vi "Meas Proc QWTB Fix Result Table Selection.vi"(7 "param table ref":refnum<vi>, 8 "error in":errorcluster) -> (0 "error out":errorcluster)   [LabVIEW 2013]
doc: "Detects position of the curcor in the table and sets selection to whole row accordingly."
uses:
  <vilib>/Utility/miscctls.llb/LVRowAndColumnTypeDef.ctl
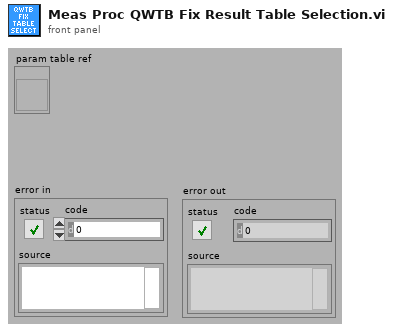
[diagram p1: front panel]
types:
  T1 = typedef "LVRowAndColumnTypeDef.ctl" = cluster{"Row":i32, "Column":i32}
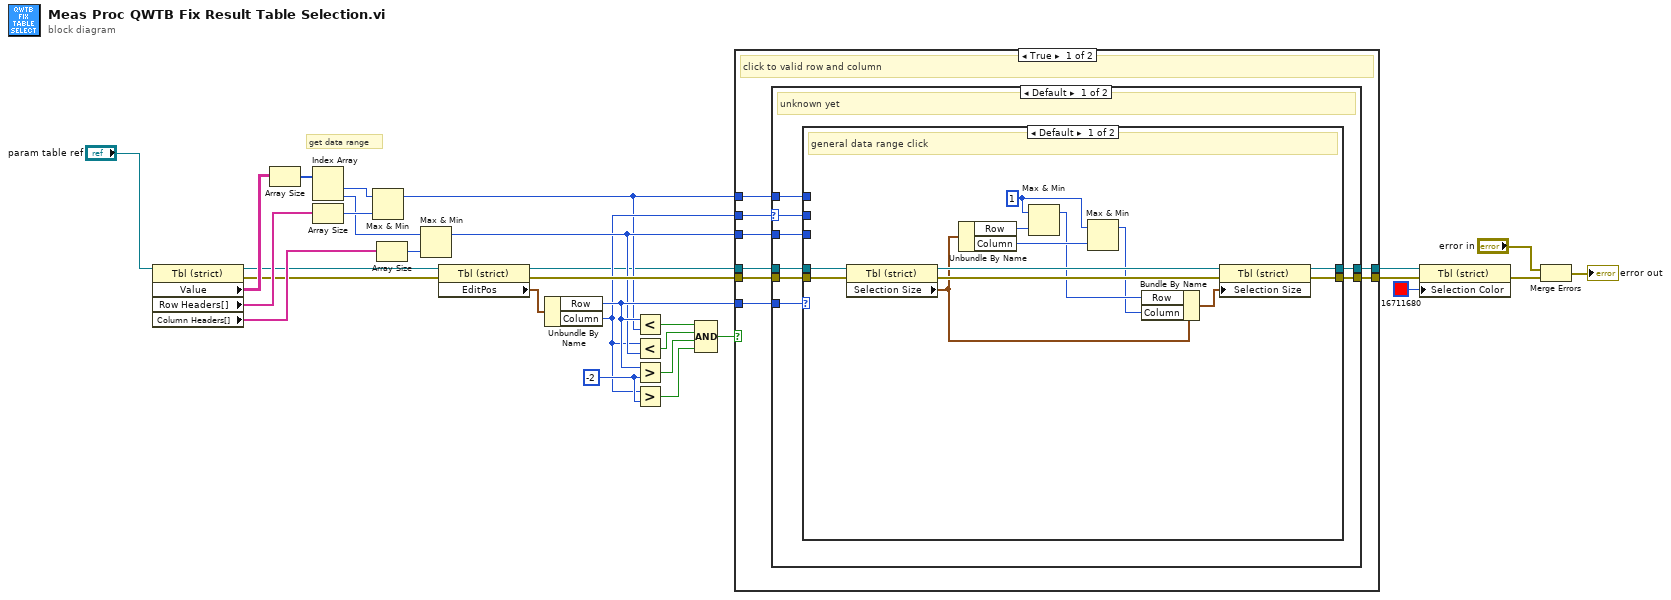
[diagram p0: block diagram]
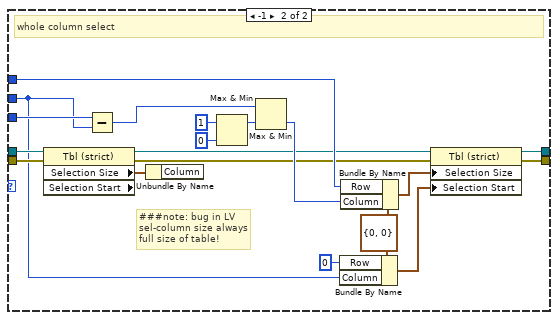
[diagram p2: hidden frame]
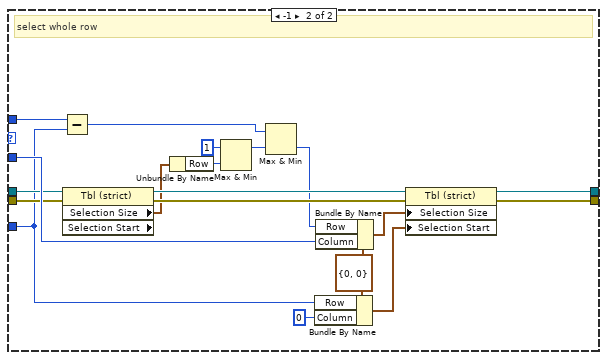
[diagram p3: hidden frame]
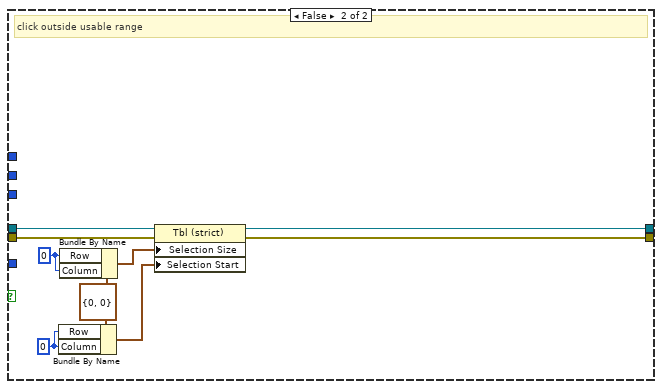
[diagram p4: hidden frame]
diagram:
  w10 = -2 ("y")
  # "get data range"
  n1 = property class="Tbl (strict)"(reference="param table ref") -> (reference out=w21:refnum<vi>, error out=w19:errorcluster, "Value"=w28:string[][], "Row Headers[]"=w26:string[], "Column Headers[]"=w22:string[])  [unwired: 1 in]
  n2 = Array Size(array=w28) -> (size(s)=w27:i32[])
  n3 = Index Array(array=w27) -> (element #1=w3:i32, element #2=w2:i32)  [unwired: 2 in]
  n4 = Array Size(array=w26) -> (size(s)=w25:i32)
  n5 = Max & Min(x=w3, y=w25) -> (max(x,y)=w4:i32)  [unwired: 1 out]
  n6 = Array Size(array=w22) -> (size(s)=w23:i32)
  n7 = Max & Min(x=w2, y=w23) -> (max(x,y)=w6:i32)  [unwired: 1 out]
  n8 = property class="Tbl (strict)"(reference=w21, error in=w19) -> (reference out=w1:refnum<vi>, error out=w18:errorcluster, "EditPos"=w20:T1)
  n9 = Unbundle By Name(w20) -> ("Row"=w11:i32, "Column"=w5:i32)
  n10 = Less?(x=w11, y=w4) -> (x < y?=w13:bool)
  n11 = Less?(x=w5, y=w6) -> (x < y?=w12:bool)
  n12 = Greater?(x=w11, y=w10) -> (0:w9:bool)
  n13 = Greater?(x=w5, y=w10) -> (0:w8:bool)
  n14 = Compound Arithmetic op=AND(w13, w12, w9, w8) -> (w7:bool)
  n15 = case shown="True" w7 {
    tunnel: w18 -> [w38 w106]
    tunnel: w1 -> [w37 w105]
    tunnel: w11 -> [w33 _]
    tunnel: w6 -> [w36 _]
    tunnel: [w35 w101] -> w17
    tunnel: [w34 w100] -> w16
    tunnel: w5 -> [w32 _]
    tunnel: w4 -> [w31 _]
    frame True {
      # "click to valid row and column"
      n16 = case shown="Default" w32 {
        selector: w32 -> [w40 _]
        tunnel: w38 -> [w46 w90]
        tunnel: w37 -> [w45 w89]
        tunnel: w36 -> [w44 w96]
        tunnel: [w43 w92] -> w35
        tunnel: [w42 w91] -> w34
        tunnel: w33 -> [w41 w82]
        tunnel: w31 -> [w39 w83]
        frame Default {
          # "unknown yet"
          n17 = case shown="Default" w41 {
            tunnel: w46 -> [w59 w72]
            tunnel: w45 -> [w58 w71]
            tunnel: w44 -> [_ w70]
            tunnel: [w55 w74] -> w43
            tunnel: [w54 w73] -> w42
            tunnel: w40 -> [_ w65]
            tunnel: w39 -> [_ w63]
            frame Default {
              w51 = 1 ("x")
              # "general data range click"
              n18 = property class="Tbl (strict)"(reference=w58, error in=w59) -> (reference out=w56:refnum<vi>, error out=w57:errorcluster, "Selection Size"=w50:T1)
              n19 = Unbundle By Name(w50) -> ("Row"=w53:i32, "Column"=w52:i32)
              n20 = Max & Min(x=w51, y=w53) -> (max(x,y)=w49:i32)  [unwired: 1 out]
              n21 = Max & Min(x=w51, y=w52) -> (max(x,y)=w48:i32)  [unwired: 1 out]
              n22 = Bundle By Name(cluster=w50, "Row"=w49, "Column"=w48) -> (w47:T1)
              n23 = property class="Tbl (strict)"(reference=w56, error in=w57, "Selection Size"=w47) -> (reference out=w54:refnum<vi>, error out=w55:errorcluster)
            }
            frame -1 {
              w77 = T1 {"Row"=0, "Column"=0} ("Selection Size")
              # "###note: bug in LV\nsel-column size always \nfull size of table!"
              # "whole column select"
              n24 = property class="Tbl (strict)" props=["Selection Size", "Selection Start"](reference=w71, error in=w72) -> (reference out=w61:refnum<vi>, error out=w62:errorcluster, "Selection Size"=w69:T1)  [unwired: 1 out]
              n25 = Subtract(x=w70, y=w65) -> (x-y=w66:i32)
              n26 = Unbundle By Name(w69) -> ()  [unwired: 1 out]
              n27 = Max & Min(x=1, y=0) -> (max(x,y)=w67:i32)  [unwired: 1 out]
              n28 = Max & Min(x=w66, y=w67) -> (min(x,y)=w64:i32)  [unwired: 1 out]
              n29 = Bundle By Name(cluster=w77, "Row"=0 ("Column"), "Column"=w65) -> (w76:T1)
              n30 = Bundle By Name(cluster=w77, "Row"=w63, "Column"=w64) -> (w78:T1)
              n31 = property class="Tbl (strict)"(reference=w61, error in=w62, "Selection Size"=w78, "Selection Start"=w76) -> (reference out=w73:refnum<vi>, error out=w74:errorcluster)
            }
          }
        }
        frame -1 {
          w95 = T1 {"Row"=0, "Column"=0} ("Selection Size")
          # "select whole row"
          n32 = Subtract(x=w83, y=w82) -> (x-y=w80:i32)
          n33 = property class="Tbl (strict)" props=["Selection Size", "Selection Start"](reference=w89, error in=w90) -> (reference out=w87:refnum<vi>, error out=w88:errorcluster, "Selection Size"=w86:T1)  [unwired: 1 out]
          n34 = Unbundle By Name(w86) -> ("Row"=w85:i32)
          n35 = Max & Min(x=1, y=w85) -> (max(x,y)=w81:i32)  [unwired: 1 out]
          n36 = Max & Min(x=w80, y=w81) -> (min(x,y)=w79:i32)  [unwired: 1 out]
          n37 = Bundle By Name(cluster=w95, "Row"=w82, "Column"=0) -> (w94:T1)
          n38 = Bundle By Name(cluster=w95, "Row"=w79, "Column"=w96) -> (w97:T1)
          n39 = property class="Tbl (strict)"(reference=w87, error in=w88, "Selection Size"=w97, "Selection Start"=w94) -> (reference out=w91:refnum<vi>, error out=w92:errorcluster)
        }
      }
    }
    frame False {
      w98 = 0 ("Column")
      w99 = 0 ("Row")
      w103 = T1 {"Row"=0, "Column"=0} ("Selection Size")
      # "click outside usable range"
      n40 = Bundle By Name(cluster=w103, "Row"=w98, "Column"=w98) -> (w102:T1)
      n41 = Bundle By Name(cluster=w103, "Row"=w99, "Column"=w99) -> (w104:T1)
      n42 = property class="Tbl (strict)"(reference=w105, error in=w106, "Selection Size"=w104, "Selection Start"=w102) -> (reference out=w100:refnum<vi>, error out=w101:errorcluster)
    }
  }
  n43 = property class="Tbl (strict)"(reference=w16, error in=w17, "Selection Color"=u32 16711680) -> (error out=w14:errorcluster)  [unwired: 1 out]
  n44 = Merge Errors("error in", w14) -> (→"error out":errorcluster)
